vi "setCurrentOutputState.vi"(8 "error in (no error)":errorcluster, 9 "CurrentOutputState":T1(array[cluster]), 10 "CurrentChannels":string[](array[string]), 11 "DDSOutput in":refnum<class "DDSOutput.lvclass">) -> (0 "error out":errorcluster, 3 "DDSOutput out":refnum<class "DDSOutput.lvclass">)   [LabVIEW 2009, in "Hardware.lvlib" / "Channels.lvlib" / "DDSOutput.lvclass"]
uses:
  DDSOutput.lvclass
  DDSOutput.lvclass/DDSOutput.ctl
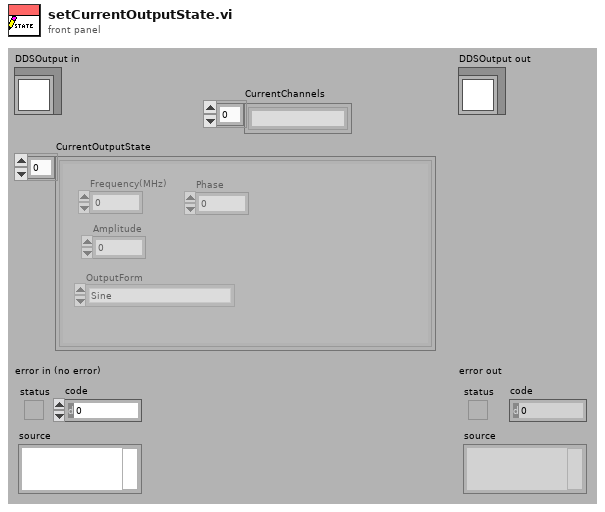
[diagram p1: front panel]
types:
  T1 = cluster{"Frequency(MHz)":dbl, "Amplitude":dbl, "Phase":dbl, "OutputForm":enum16{"Sine", "Square", "Triangle", "Arbitrary"}}[]
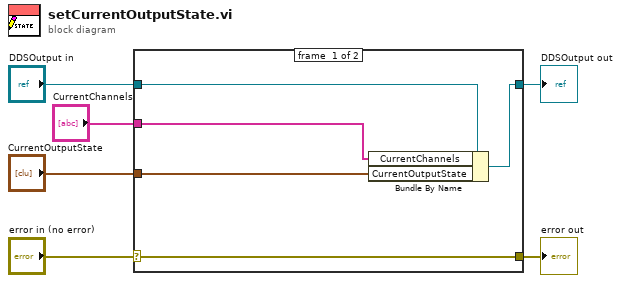
[diagram p0: block diagram]
diagram:
  n1 = case shown="No Error" "error in (no error)" {
    selector: "error in (no error)" -> [w11 w12]
    tunnel: [w11 w12] -> w5
    tunnel: [w9 w13] -> w3
    tunnel: "DDSOutput in" -> [w10 w13]
    tunnel: "CurrentOutputState" -> [w8 _]
    tunnel: "CurrentChannels" -> [w7 _]
    frame #0 {
      n2 = Bundle By Name(cluster=w10, "CurrentChannels"=w7, "CurrentOutputState"=w8) -> (w9:refnum<class "DDSOutput.lvclass">)
    }
    frame #1 {
    }
  }
  "error out" <- w5
  "DDSOutput out" <- w3
